vi "get backslash codes text.vi"(10 "error in (no error)":errorcluster, 11 "String in":refnum<vi>) -> (0 "normal text":string, 1 "'\\' codes text":string, 2 "error out":errorcluster, 3 "String in 2":refnum<vi>)   [LabVIEW 2018]
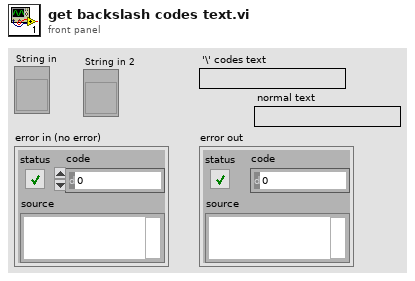
[diagram p1: front panel]
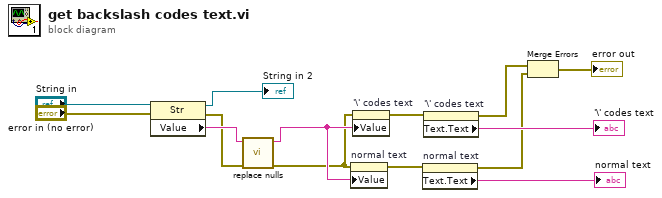
[diagram p0: block diagram]
diagram:
  n1 = property class="Str"(reference="String in", error in="error in (no error)") -> (reference out=→"String in 2":refnum<vi>, error out=w2:errorcluster, "Value"=w4:string)
  n2 = call "replace nulls.vi"("error in (no error)"=w2, "read buffer"=w4) -> ("error out"=w1:errorcluster, "result string"=w3:string)  [unwired: 8 in]
  n3 = property on="normal text" class="Str"(error in=w1, "Value"=w3) -> (error out=w11:errorcluster)  [unwired: 1 in, 1 out]
  n4 = property on="'\\' codes text" class="Str"(error in=w1, "Value"=w3) -> (error out=w12:errorcluster)  [unwired: 1 in, 1 out]
  n5 = property on="normal text" class="Str"(error in=w11) -> (error out=w6:errorcluster, "Text.Text"=→"normal text":string)  [unwired: 1 in, 1 out]
  n6 = property on="'\\' codes text" class="Str"(error in=w12) -> (error out=w7:errorcluster, "Text.Text"=→"'\\' codes text":string)  [unwired: 1 in, 1 out]
  n7 = Merge Errors(w7, w6) -> (→"error out":errorcluster)
